vi "Unit Test expand objects on type conflict False.vi"() -> ()   [LabVIEW 2019, in "Sports Unit Tests.lvclass"]
uses:
  Sports Unit Tests.lvclass
  Classes/Sports Player/Sports Player.lvclass
  C:/DSCE code/Serialization/blueserializationdemo/Test/Sports/Classes/Human/Human.lvclass
  Classes/Tiger Woods/Tiger Woods.lvclass
  <userlib>/Blue Origin/BlueSerialization/BlueSerializer/DeserializeOptions.ctl
  <userlib>/Blue Origin/BlueSerialization/BlueSerializer/DeserializeSlicingOptions.ctl
  <userlib>/Blue Origin/BlueSerialization/BlueSerializer/DeserializeMutationOptions.ctl
  <userlib>/Blue Origin/BlueSerialization/BlueSerializer/DeserializePreservationOptions.ctl
  <userlib>/Blue Origin/BlueSerialization/BlueSerializer/PreserveNonWiredDataOption.ctl
  Classes/Human/Human.lvclass/Human.ctl
  Classes/Sports Player/Sports Player.lvclass/Sports Player.ctl
  Classes/Human/Write Age (years).vi
  Classes/Human/Write alive_.vi
  Classes/Human/Write Height (ft).vi
  Classes/Human/Write Name.vi
  Classes/Sports Player/Write Earnings (dollars).vi
  Classes/Sports Player/Write Professional_.vi
  Classes/Sports Player/Write Sponsor.vi
  <vilib>/Utility/error.llb/Clear Errors.vi
  <vilib>/addons/_JKI Toolkits/Caraya/classes/Test/Define Test.vi
  <vilib>/addons/_JKI Toolkits/Caraya/classes/Assert/Assert Equal Value_Variant.vi
  <vilib>/addons/_JKI Toolkits/Caraya/classes/Assert/Assert Error.vi
  <vilib>/addons/_JKI Toolkits/Caraya/classes/Assert/Assert.lvclass
  <userlib>/Blue Origin/BlueSerialization/BlueSerializer/BlueSerializer.lvclass
panel:
  out "Table":string[][](table)
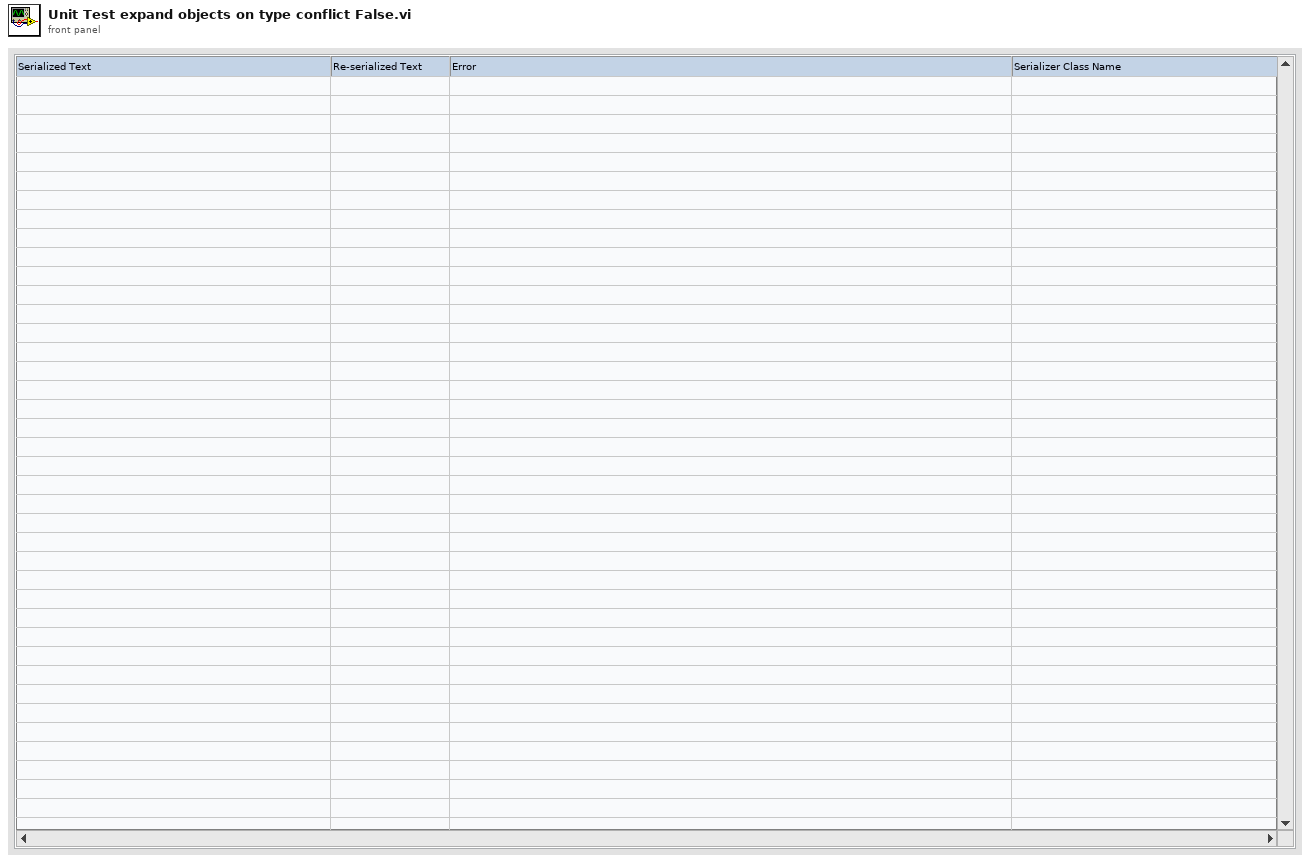
[diagram p1: front panel]
types:
  T1 = typedef "BlueSerialization.lvlib/BlueSerializer.lvclass/DeserializeOptions.ctl" = cluster{"deserialize non-BlueSerializable objects from hex?":bool, "expand objects on type conflict?":bool, "Slicing":T2, "Mutation Options":T3, "Preservation Options":T4}
  T2 = typedef "BlueSerialization.lvlib/BlueSerializer.lvclass/DeserializeSlicingOptions.ctl" = cluster{"slice flattened object data on error?":bool, "sliceable class names":string[]}
  T3 = typedef "BlueSerialization.lvlib/BlueSerializer.lvclass/DeserializeMutationOptions.ctl" = cluster{"error on inserted parent levels?":bool, "\terror on obsolete parent levels?":bool}
  T4 = typedef "BlueSerialization.lvlib/BlueSerializer.lvclass/DeserializePreservationOptions.ctl" = cluster{"Preserve wired serialized data?":bool, "Preserve wired non-serialized data":T5}
  T5 = typedef "BlueSerialization.lvlib/BlueSerializer.lvclass/PreserveNonWiredDataOption.ctl" = enum16{"Don't preserve", "Preserve (error on less-specific wired types)", "Preserve (except on less-specific wired types)"}
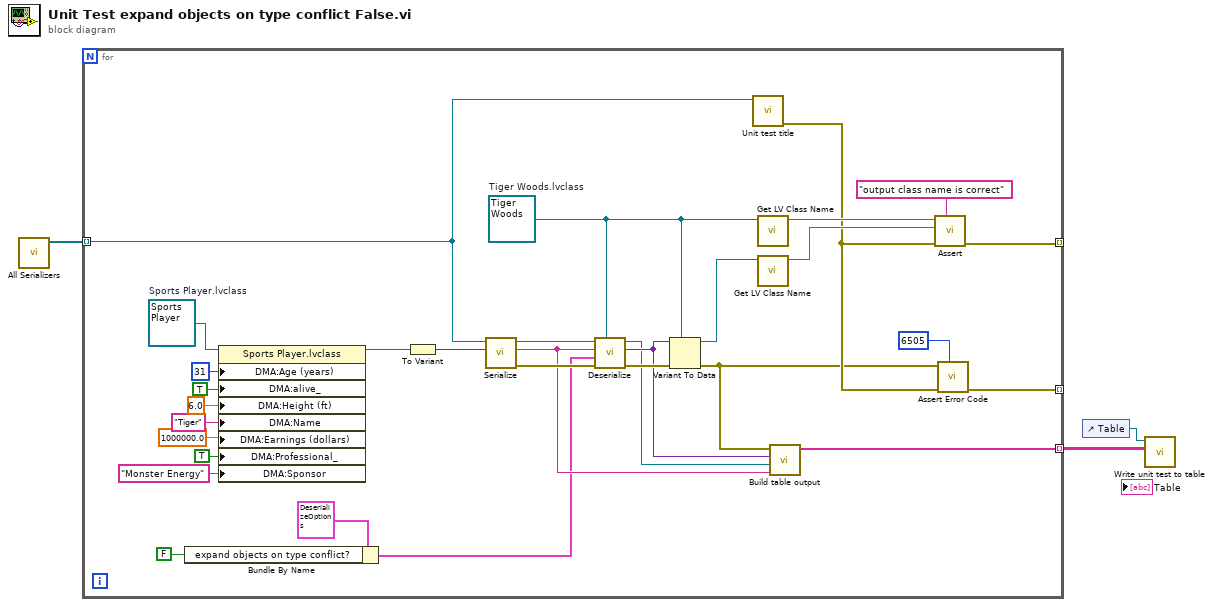
[diagram p0: block diagram]
diagram:
  n1 = call "All Serializers.vi"() -> ("All serializers"=w2:refnum<class "BlueSerializer.lvclass">[])  [unwired: 11 in]
  n2 = for {
    tunnel: w2 -> [w5] mode=indexing
    tunnel: [w15] -> _ mode=indexing
    tunnel: [w16] -> _ mode=indexing
    tunnel: [w8] -> w1 mode=indexing
    w17 = refnum<class "Tiger Woods.lvclass"> refnum  # Tiger Woods.lvclass
    w26 = refnum<class "Sports Player.lvclass"> refnum  # Sports Player.lvclass
    n3 = Bundle By Name(cluster=T1 {"deserialize non-BlueSerializable objects from hex?"=FALSE, "expand objects on type conflict?"=FALSE, "Slicing"={"slice flattened object data on error?"=FALSE, "sliceable class names"=[]}, "Mutation Options"={"error on inserted parent levels?"=FALSE, "\terror on obsolete parent levels?"=FALSE}, "Preservation Options"={"Preserve wired serialized data?"=FALSE, "Preserve wired non-serialized data"=enum."Don't preserve"}} ("Deserialize Options"), "expand objects on type conflict?"=FALSE ("Allow class expansion?")) -> (w4:T1)
    n4 = property on="Property Node" class="Sports Player.lvclass"(reference=w26, "DMA:Age (years)"=u16 31 ("Age (years)"), "DMA:alive_"=TRUE ("alive_"), "DMA:Height (ft)"=6.0 ("Height (ft)"), "DMA:Name"="Tiger" ("Name"), "DMA:Earnings (dollars)"=1000000.0 ("Earnings (dollars)"), "DMA:Professional_"=TRUE ("Professional_"), "DMA:Sponsor"="Monster Energy" ("Sponsor")) -> (reference out=w18:refnum<class "Sports Player.lvclass">)  [unwired: 1 in, 1 out]
    n5 = To Variant(anything=w18) -> (Variant=w32:variant)
    n6 = call <userlib>:"Serialize.vi"("Anything"=w32, "BlueSerializer in"=w5) -> ("error out"=w34:errorcluster, "Serialized Text"=w9:string, "BlueSerializer out"=w33:refnum<class "BlueSerializer.lvclass">)  [unwired: 7 in]
    n7 = call <userlib>:"Deserialize.vi"("Anything"=w17, "error in (no error)"=w34, "Deserialize Options"=w4, "Serialized Text"=w9, "BlueSerializer in"=w33) -> ("error out"=w31:errorcluster, "Variant"=w11:variant, "BlueSerializer out"=w10:refnum<class "BlueSerializer.lvclass">)  [unwired: 4 in]
    n8 = Variant To Data(error in=w31, type=w17, Variant=w11) -> (data=w30:refnum<class "Tiger Woods.lvclass">, error out=w12:errorcluster)
    n9 = call "Unit test title.vi"("serializer"=w5) -> ("error out"=w13:errorcluster)  [unwired: 9 in, 1 out]
    n10 = call <vilib>:"Get LV Class Name.vi"("object"=w17) -> ("class name"=w29:string)  [unwired: 9 in, 1 out]
    n11 = call <vilib>:"Get LV Class Name.vi"("object"=w30) -> ("class name"=w28:string)  [unwired: 9 in, 1 out]
    n12 = call "Build table output.vi"("serialized text"=w9, "BlueSerializer in"=w10, "deserialized variant"=w11, "variant to data error"=w12) -> ("table output"=w8:string[])  [unwired: 7 in]
    n13 = call-poly <vilib>:"Assert.vi"("Label"="output class name is correct", "error in (no error)"=w13, "Y"=w28, "X"=w29) -> ("error out"=w16:errorcluster)  [unwired: 7 in]
    n14 = call "Assert Error Code.vi"("Assert specific error code"=6505 ("error code (1)"), "error in (no error)"=w13, "Error?"=w12) -> ("error out"=w15:errorcluster)  [unwired: 8 in]
  }
  n15 = control-ref of="Table"() -> (w3:refnum<vi>)
  n16 = call "Write unit test to table.vi"("Table"=w1, "Table ref in"=w3) -> ()  [unwired: 9 in, 1 out]
